vi "record_line (SubVI).vi"(7 "topo_pixel":i32, 8 "error in (no error)":errorcluster, 9 "Data_in":dbl[][][](array[numeric]), 10 "Settings in":T1, 11 "Application in":refnum<vi>) -> (0 "error out":errorcluster, 1 "Data_out":sgl[][][](array[numeric]), 3 "Application out":refnum<vi>)   [LabVIEW 2014]
uses:
  <userlib>/Nanonis Prog Interface V5/Nanonis Prog Interface.lvlib
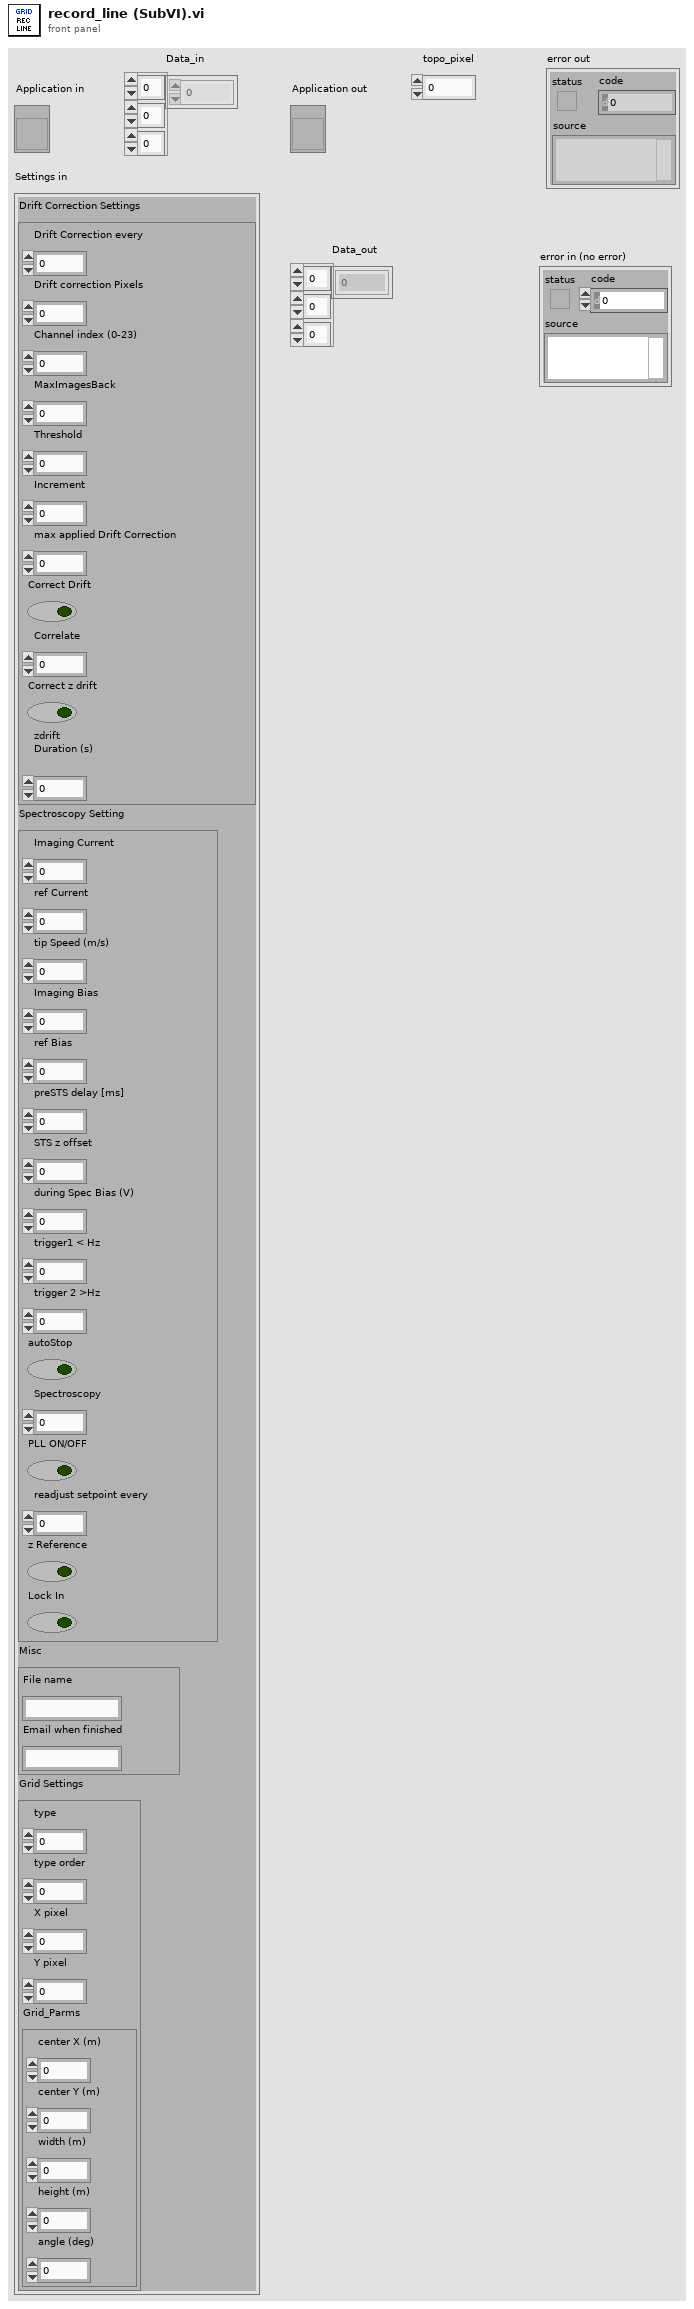
[diagram p1: front panel]
types:
  T1 = cluster{"Drift Correction Settings":cluster{"Drift Correction every":i32, "Drift correction Pixels":i32, "Channel index (0-23)":u8, "MaxImagesBack":i32, "Threshold":i32, "Increment":i32, "max applied Drift Correction":i32, "Correct Drift":bool, "Correlate":u16, "Correct z drift":bool, "zdrift \nDuration (s)":dbl}, "Spectroscopy Setting":cluster{"Imaging Current":dbl, "ref Current":dbl, "tip Speed (m/s)":sgl, "Imaging Bias":dbl, "ref Bias":dbl, "preSTS delay [ms]":u32, "STS z offset":dbl, "during Spec Bias (V)":sgl, "trigger1 < Hz":sgl, "trigger 2 >Hz":sgl, "autoStop":bool, "Spectroscopy":u16, "PLL ON/OFF":bool, "readjust setpoint every ":i32, "z Reference":bool, "Lock In":bool}, "Misc":cluster{"File name":string, "Email when finished":string}, "Grid Settings":cluster{"type":u16, "type order":u16, "X pixel":i32, "Y pixel":i32, "Grid_Parms":cluster{"center X (m)":sgl, "center Y (m)":sgl, "width (m)":sgl, "height (m)":sgl, "angle (deg)":sgl}}}
  T2 = cluster{"type":u16, "type order":u16, "X pixel":i32, "Y pixel":i32, "Grid_Parms":cluster{"center X (m)":sgl, "center Y (m)":sgl, "width (m)":sgl, "height (m)":sgl, "angle (deg)":sgl}}
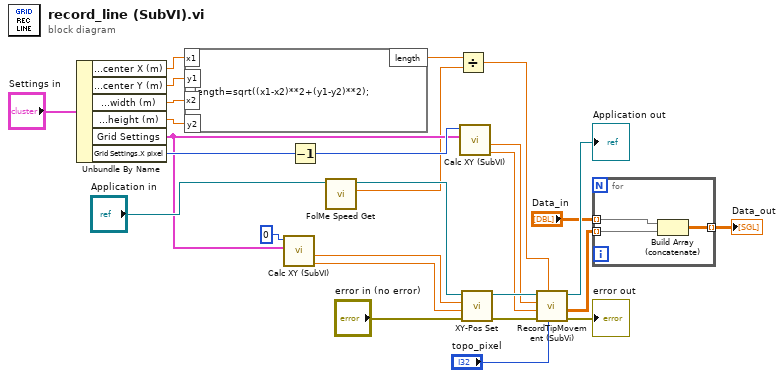
[diagram p0: block diagram]
diagram:
  n1 = Unbundle By Name("Settings in") -> ("Grid Settings.Grid_Parms.center X (m)"=w8:sgl, "Grid Settings.Grid_Parms.center Y (m)"=w7:sgl, "Grid Settings.Grid_Parms.width (m)"=w6:sgl, "Grid Settings.Grid_Parms.height (m)"=w1:sgl, "Grid Settings"=w9:T2, "Grid Settings.X pixel"=w10:i32)
  n2 = formula code="length=sqrt((x1-x2)**2+(y1-y2)**2);"("x1"=w8, "x2"=w6, "y1"=w7, "y2"=w1) -> ("length"=w5:dbl)
  n3 = call "Calc XY (SubVI).vi"("Grid Settings"=w9, "element"=i64 0) -> ("y2"=w25:dbl, "x2"=w24:dbl)  [unwired: 6 in, 2 out]
  n4 = Decrement(x=w10) -> (x-1=w27:i32)
  n5 = call <userlib>:"FolMe Speed Get.vi"("Application ref in"="Application in") -> ("Speed (m/s)"=w4:sgl, "Application ref out"=w11:refnum<vi>)  [unwired: 5 in, 2 out]
  n6 = Divide(x=w5, y=w4) -> (x/y=w3:dbl)
  n7 = call "Calc XY (SubVI).vi"("Grid Settings"=w9, "element"=w27) -> ("y2"=w22:dbl, "x2"=w21:dbl)  [unwired: 6 in, 2 out]
  n8 = call <userlib>:"XY-Pos Set.vi"("error in (no error)"="error in (no error)", "Y (m)"=w25, "X (m)"=w24, "Application ref in"=w11) -> ("error out"=w18:errorcluster, "Application ref out"=w26:refnum<vi>)  [unwired: 4 in]
  n9 = call "RecordTipMovement (SubVi).vi"("Pixel"="topo_pixel", "time"=w3, "error in (no error)"=w18, "Y (m)"=w22, "X (m)"=w21, "Application ref in"=w26) -> ("error out"=→"error out":errorcluster, "Data"=w14:sgl[][], "Application ref out"=→"Application out":refnum<vi>)  [unwired: 2 in, 1 out]
  n10 = for {
    tunnel: w14 -> [w28] mode=indexing
    tunnel: "Data_in" -> [w30] mode=indexing
    tunnel: [w29] -> w13 mode=indexing
    n11 = Build Array (concatenate)(w30, w28) -> (w29:dbl[][])
  }
  "Data_out" <- w13
